vi "Read Lock Boolean Text.vi"(9 "Boolean in":refnum<class "Boolean.lvclass">) -> (3 "Boolean out":refnum<class "Boolean.lvclass">, 4 "Lock Boolean Text":bool)   [LabVIEW 2014, in "Boolean.lvclass"]
uses:
  Boolean.lvclass
  Boolean.lvclass/Boolean.ctl
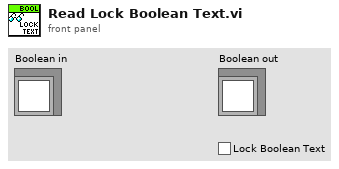
[diagram p1: front panel]
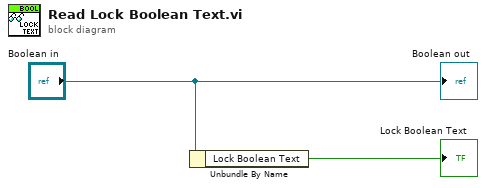
[diagram p0: block diagram]
diagram:
  n1 = Unbundle By Name("Boolean in") -> ("Lock Boolean Text"=→"Lock Boolean Text":bool)
  "Boolean out" <- "Boolean in"
